vi "Send RX Message.vi"(8 "error in (no error)":errorcluster, 11 "RxTx in":refnum<class "RxTx.lvclass">) -> (0 "error out":errorcluster, 3 "RxTx out":refnum<class "RxTx.lvclass">)   [LabVIEW 2018, in "RxTx.lvclass"]
uses:
  RxTx.lvclass
  RxTx.lvclass/RxTx.ctl
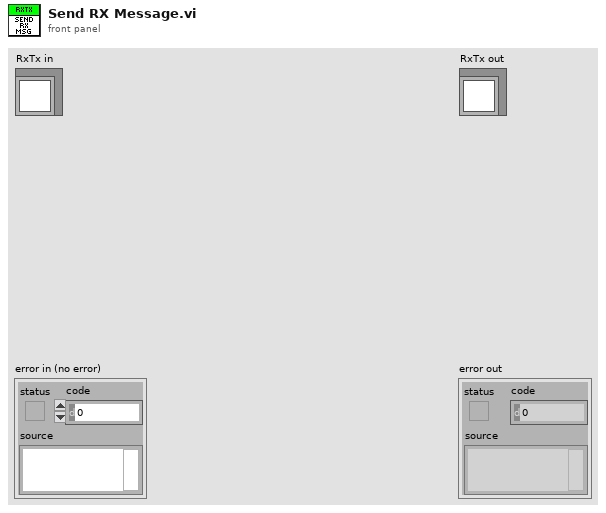
[diagram p1: front panel]
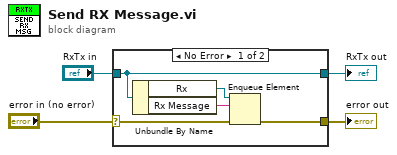
[diagram p0: block diagram]
diagram:
  n1 = case shown="No Error" "error in (no error)" {
    selector: "error in (no error)" -> [w8 w11]
    tunnel: [w9 w11] -> w2
    tunnel: [w6 w10] -> w1
    tunnel: "RxTx in" -> [w6 w10]
    frame No Error {
      n2 = Unbundle By Name(w6) -> ("Rx"=w7:refnum<queue>, "Rx Message"=w5:string)
      n3 = Enqueue Element(queue=w7, element=w5, error in (no error)=w8) -> (error out=w9:errorcluster)  [unwired: 1 in, 2 out]
    }
    frame Error {
    }
  }
  "error out" <- w2
  "RxTx out" <- w1
